vi "iPSread.vi"(8 "error in (no error)":errorcluster, 10 "iPSreadCtrl":T1=enum."Switch Heater Temp", 11 "VISA resource name":refnum<visa-resource-name>) -> (0 "error out":errorcluster, 1 "read buffer":string, 2 "number":dbl, 3 "VISA resource name out":refnum<visa-resource-name>)   [LabVIEW 2017]
uses:
  controls/iPSreadCtrl.ctl
  <vilib>/regexp/Match Regular Expression.xnode
panel:
  out "after match":string
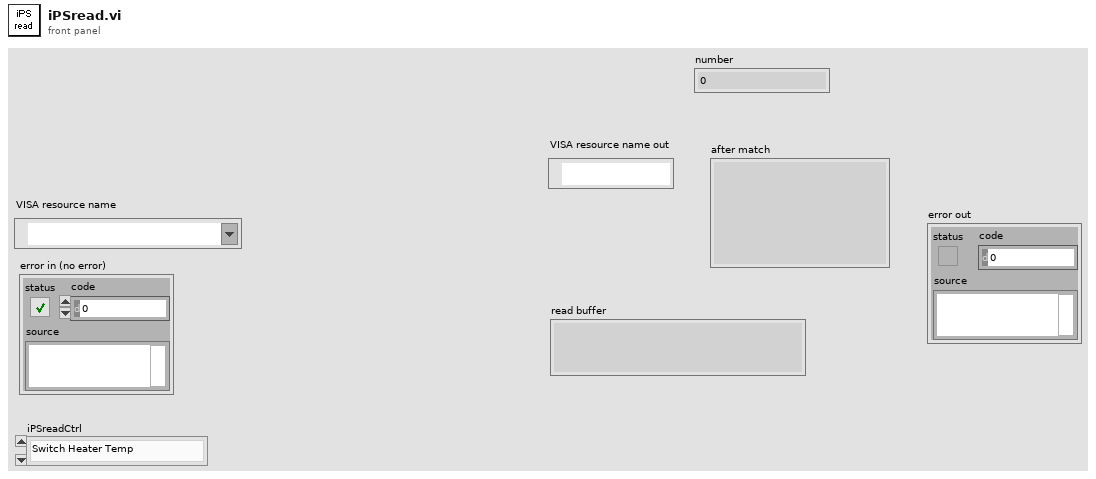
[diagram p1: front panel]
types:
  T1 = typedef "iPSreadCtrl.ctl" = enum16{"OutputField", "MagnetField", "Switch Heater Temp", "Field Rate", "Magnet Temp"}
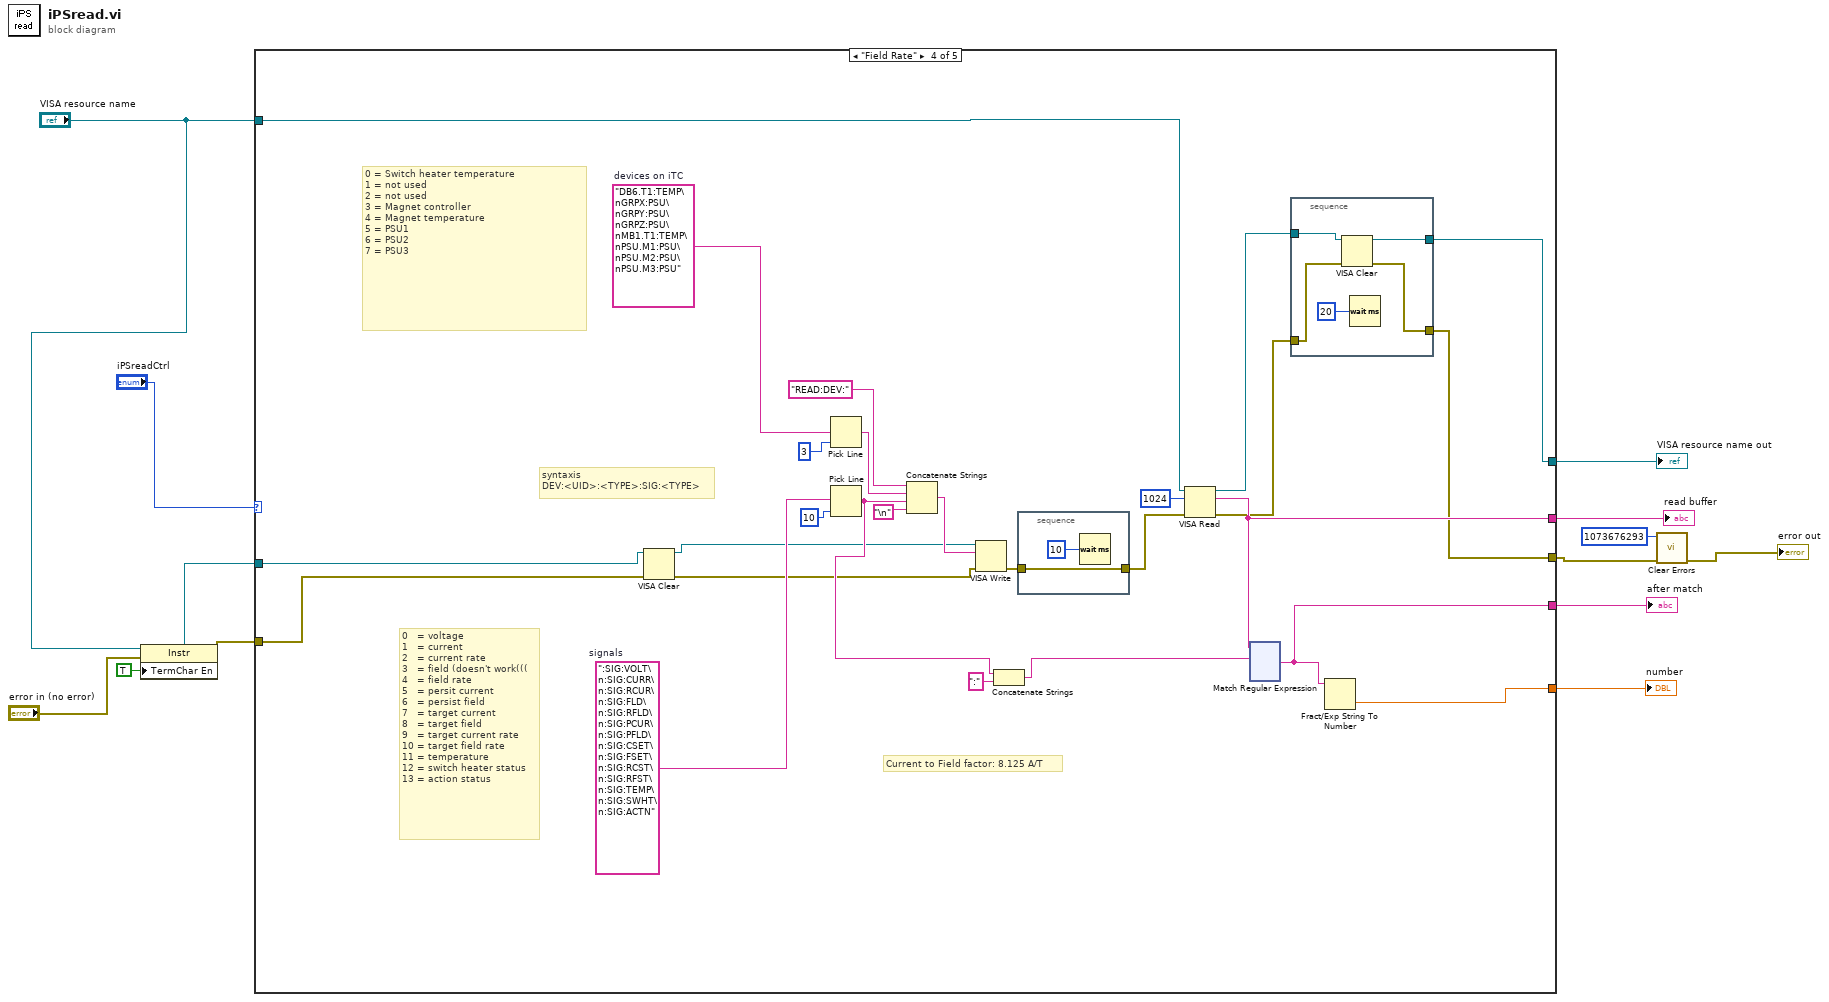
[diagram p0: block diagram]
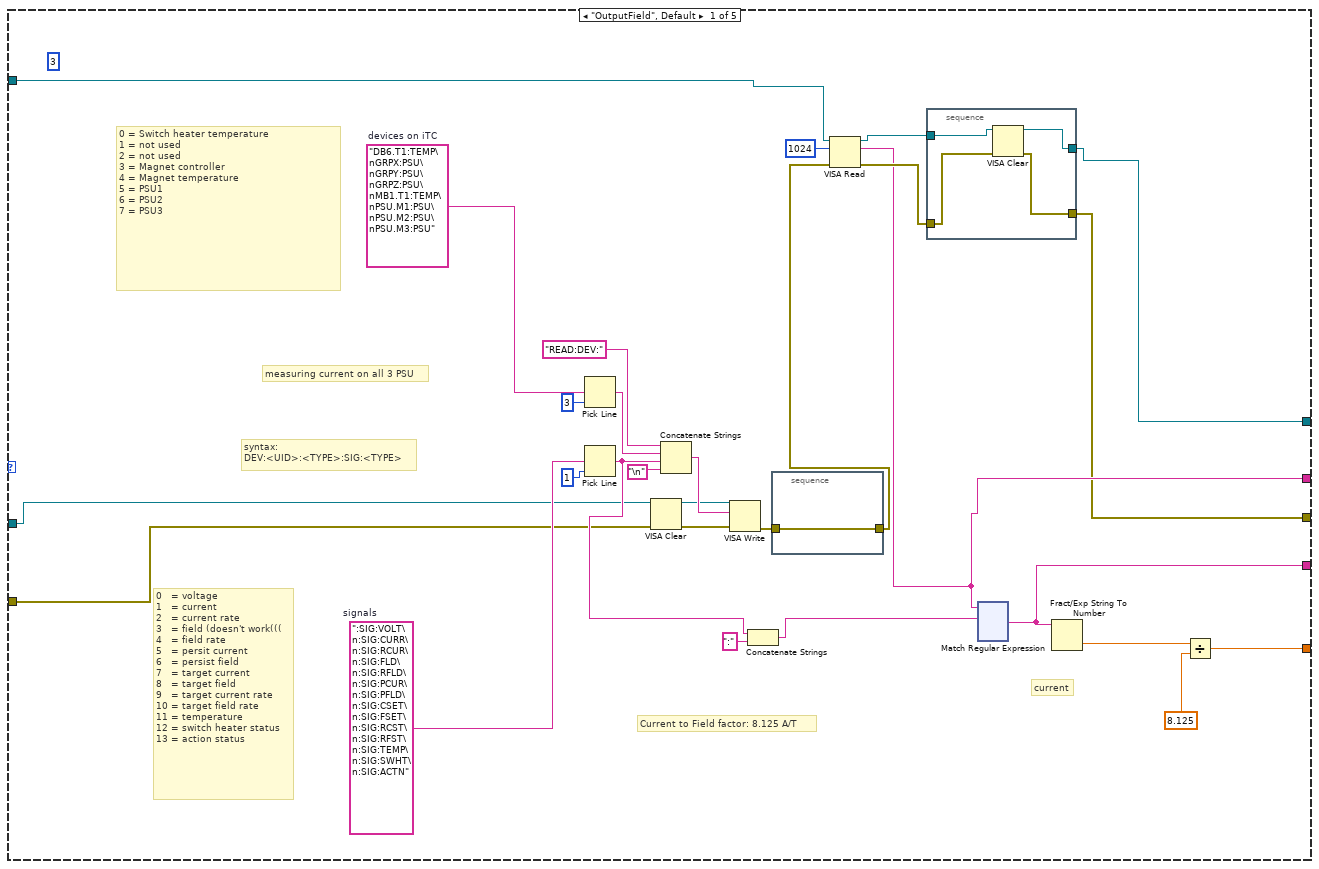
[diagram p2: hidden frame]
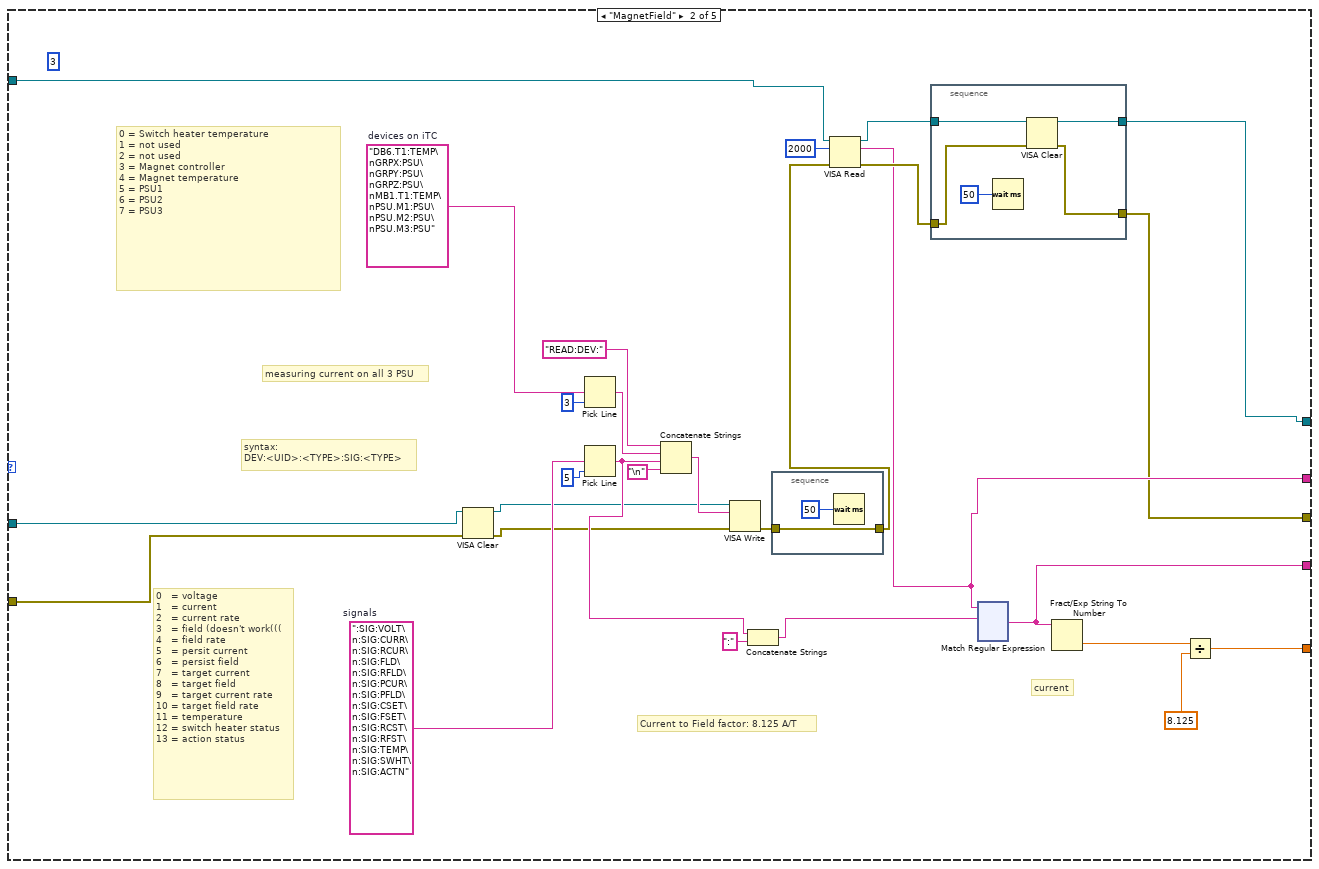
[diagram p3: hidden frame]
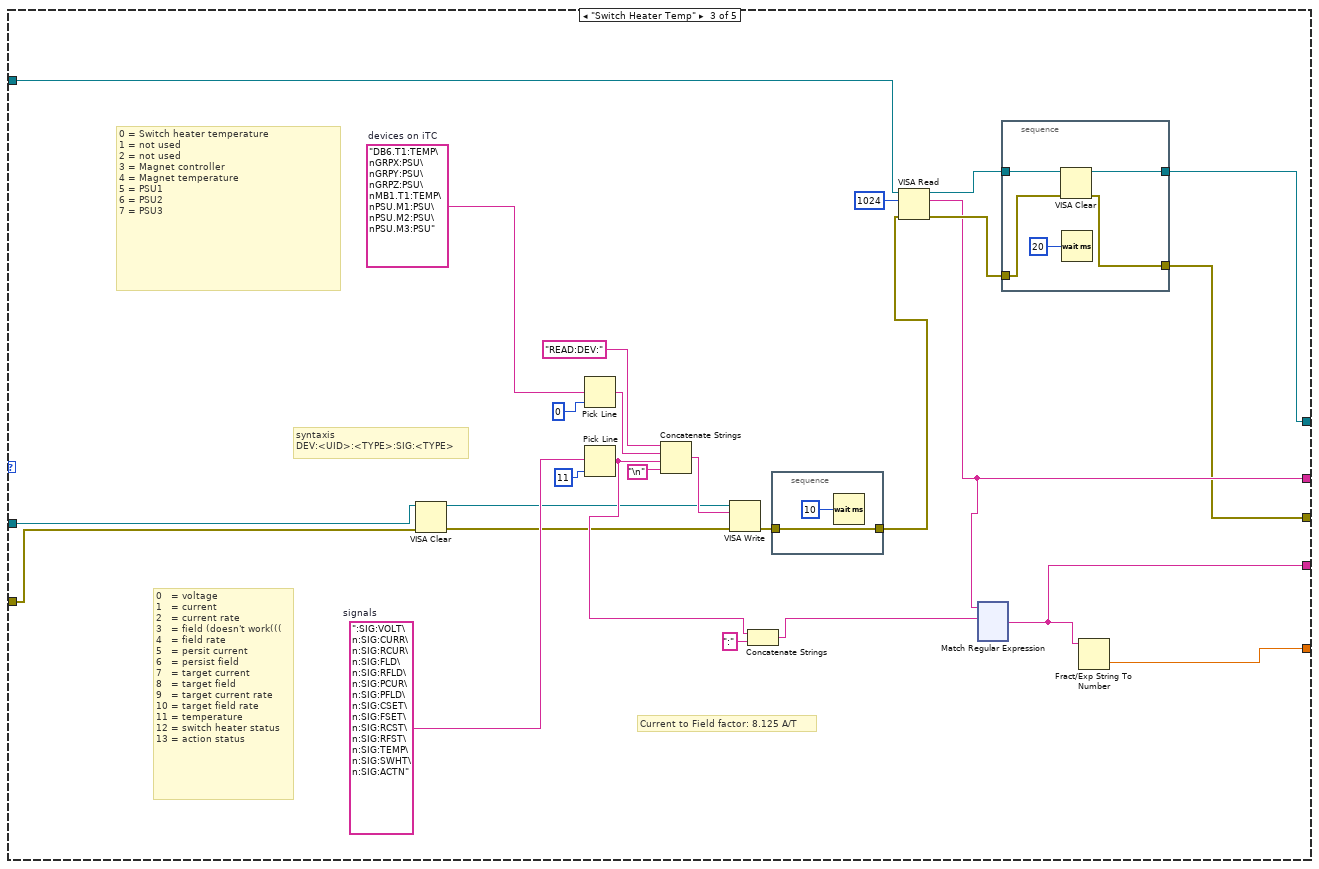
[diagram p4: hidden frame]
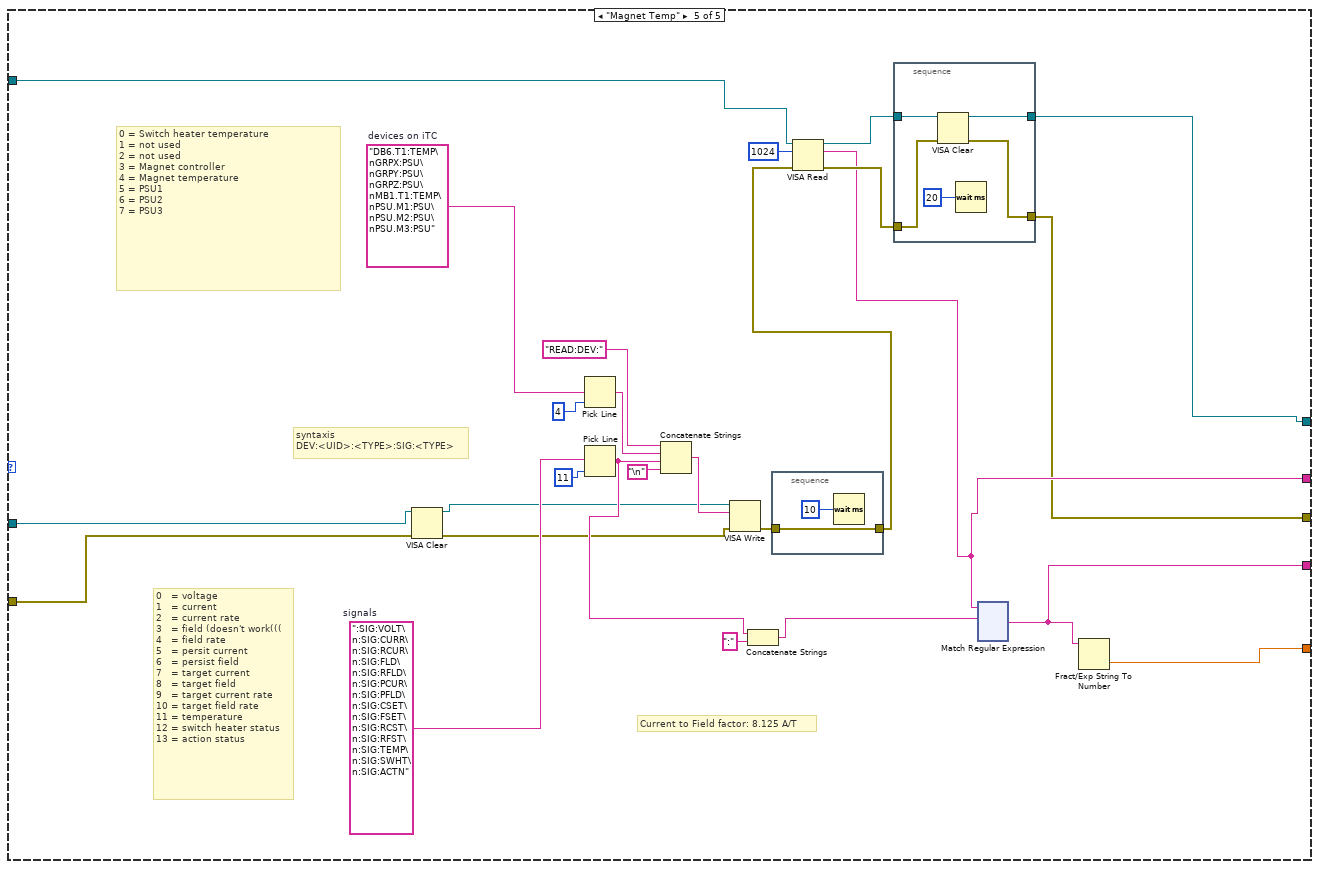
[diagram p5: hidden frame]
diagram:
  n1 = property class="Instr"(reference="VISA resource name", error in="error in (no error)", "TermChar En"=TRUE ("Message Based Settings:Termination Character Enable")) -> (reference out=w7:refnum<visa-resource-name>, error out=w5:errorcluster)
  n2 = case shown="\"Field Rate\"" "iPSreadCtrl" {
    tunnel: "VISA resource name" -> [w20 w164 w310 w454 w601]
    tunnel: [w21 w165 w311 w455 w598] -> w3
    tunnel: [w14 w158 w305 w448 w593] -> w13
    tunnel: [w22 w166 w313 w458 w599] -> w12
    tunnel: [w41 w185 w319 w463 w607] -> w11
    tunnel: [w39 w183 w318 w462 w606] -> w10
    tunnel: w5 -> [w18 w160 w306 w452 w594]
    tunnel: w7 -> [w19 w161 w307 w453 w595]
    frame "OutputField", Default {
      w33 = ":SIG:VOLT\n:SIG:CURR\n:SIG:RCUR\n:SIG:FLD\n:SIG:RFLD\n:SIG:PCUR\n:SIG:PFLD\n:SIG:CSET\n:SIG:FSET\n:SIG:RCST\n:SIG:RFST\n:SIG:TEMP\n:SIG:SWHT\n:SIG:ACTN"  # signals
      w38 = "DB6.T1:TEMP\nGRPX:PSU\nGRPY:PSU\nGRPZ:PSU\nMB1.T1:TEMP\nPSU.M1:PSU\nPSU.M2:PSU\nPSU.M3:PSU"  # devices on iTC
      (unwired) 3
      # "current"
      # "measuring current on all 3 PSU"
      # "Current to Field factor: 8.125 A/T"
      # "0 = Switch heater temperature\n1 = not used\n2 = not used\n3 = Magnet controller \n4 = Magnet temperature\n5 = PSU1 \n6 = PSU2\n7 = PSU3"
      # "0   = voltage\n1   = current\n2   = current rate\n3   = field (doesn't work(((\n4   = field rate\n5   = persit current\n6   = persist field\n7   = target current\n8   = target field\n9   = target current rate\n10 = target field rate \n11 = temperature\n12 = switch heater status\n13 = action status"
      # "syntax:\nDEV:<UID>:<TYPE>:SIG:<TYPE>"
      n3 = Pick Line(multi-line string=w38, line index=3) -> (output string=w35:string)  [unwired: 1 in]
      n4 = Pick Line(multi-line string=w33, line index=1) -> (output string=w31:string)  [unwired: 1 in]
      n5 = VISA Clear(VISA resource name=w19, error in (no error)=w18) -> (VISA resource name out=w17:refnum<visa-resource-name>, error out=w16:errorcluster)
      n6 = Concatenate Strings("READ:DEV:" ("write buffer"), w35, w31, "\n") -> (w29:string)
      n7 = VISA Write(VISA resource name=w17, write buffer=w29, error in (no error)=w16) -> (error out=w37:errorcluster)  [unwired: 2 out]
      n8 = Concatenate Strings(w31, ":" ("string")) -> (w30:string)
      n9 = stacked-sequence {
        tunnel: w37 -> [w157]
        tunnel: [w157] -> w23
        frame #0 {
        }
      }
      n10 = VISA Read(VISA resource name=w20, byte count=u32 1024, error in (no error)=w23) -> (VISA resource name out=w15:refnum<visa-resource-name>, read buffer=w22:string, error out=w24:errorcluster)  [unwired: 1 out]
      n11 = stacked-sequence {
        tunnel: [w44] -> w21
        tunnel: w24 -> [w43]
        tunnel: w15 -> [w42]
        tunnel: [w45] -> w14
        frame #0 {
          n12 = VISA Clear(VISA resource name=w42, error in (no error)=w43) -> (VISA resource name out=w45:refnum<visa-resource-name>, error out=w44:errorcluster)
        }
      }
      n13 = xnode "Match Regular Expression"("input string"=w22, "regular expression"=w30) -> ("after match"=w41:string)  [unwired: 4 in, 4 out]
      n14 = Fract/Exp String To Number(string=w41) -> (number=w26:dbl)  [unwired: 3 in, 1 out]
      n15 = Divide(x=w26, y=8.125) -> (x/y=w39:dbl)
    }
    frame "MagnetField" {
      w177 = ":SIG:VOLT\n:SIG:CURR\n:SIG:RCUR\n:SIG:FLD\n:SIG:RFLD\n:SIG:PCUR\n:SIG:PFLD\n:SIG:CSET\n:SIG:FSET\n:SIG:RCST\n:SIG:RFST\n:SIG:TEMP\n:SIG:SWHT\n:SIG:ACTN"  # signals
      w182 = "DB6.T1:TEMP\nGRPX:PSU\nGRPY:PSU\nGRPZ:PSU\nMB1.T1:TEMP\nPSU.M1:PSU\nPSU.M2:PSU\nPSU.M3:PSU"  # devices on iTC
      (unwired) 3
      # "current"
      # "measuring current on all 3 PSU"
      # "Current to Field factor: 8.125 A/T"
      # "0 = Switch heater temperature\n1 = not used\n2 = not used\n3 = Magnet controller \n4 = Magnet temperature\n5 = PSU1 \n6 = PSU2\n7 = PSU3"
      # "0   = voltage\n1   = current\n2   = current rate\n3   = field (doesn't work(((\n4   = field rate\n5   = persit current\n6   = persist field\n7   = target current\n8   = target field\n9   = target current rate\n10 = target field rate \n11 = temperature\n12 = switch heater status\n13 = action status"
      # "syntax:\nDEV:<UID>:<TYPE>:SIG:<TYPE>"
      n16 = VISA Clear(VISA resource name=w161, error in (no error)=w160) -> (VISA resource name out=w163:refnum<visa-resource-name>, error out=w162:errorcluster)
      n17 = Pick Line(multi-line string=w182, line index=3) -> (output string=w179:string)  [unwired: 1 in]
      n18 = Pick Line(multi-line string=w177, line index=5) -> (output string=w175:string)  [unwired: 1 in]
      n19 = Concatenate Strings("READ:DEV:" ("write buffer"), w179, w175, "\n") -> (w173:string)
      n20 = VISA Write(VISA resource name=w163, write buffer=w173, error in (no error)=w162) -> (error out=w181:errorcluster)  [unwired: 2 out]
      n21 = Concatenate Strings(w175, ":" ("string")) -> (w174:string)
      n22 = stacked-sequence {
        tunnel: w181 -> [w303]
        tunnel: [w303] -> w167
        frame #0 {
          n23 = Wait (ms)(milliseconds to wait=u32 50) -> ()  [unwired: 1 out]
        }
      }
      n24 = VISA Read(VISA resource name=w164, byte count=u32 2000, error in (no error)=w167) -> (VISA resource name out=w159:refnum<visa-resource-name>, read buffer=w166:string, error out=w168:errorcluster)  [unwired: 1 out]
      n25 = stacked-sequence {
        tunnel: [w187] -> w165
        tunnel: w168 -> [w186]
        tunnel: w159 -> [w189]
        tunnel: [w188] -> w158
        frame #0 {
          n26 = Wait (ms)(milliseconds to wait=u32 50) -> ()  [unwired: 1 out]
          n27 = VISA Clear(VISA resource name=w189, error in (no error)=w186) -> (VISA resource name out=w188:refnum<visa-resource-name>, error out=w187:errorcluster)
        }
      }
      n28 = xnode "Match Regular Expression"("input string"=w166, "regular expression"=w174) -> ("after match"=w185:string)  [unwired: 4 in, 4 out]
      n29 = Fract/Exp String To Number(string=w185) -> (number=w170:dbl)  [unwired: 3 in, 1 out]
      n30 = Divide(x=w170, y=8.125) -> (x/y=w183:dbl)
    }
    frame "Switch Heater Temp" {
      w324 = ":SIG:VOLT\n:SIG:CURR\n:SIG:RCUR\n:SIG:FLD\n:SIG:RFLD\n:SIG:PCUR\n:SIG:PFLD\n:SIG:CSET\n:SIG:FSET\n:SIG:RCST\n:SIG:RFST\n:SIG:TEMP\n:SIG:SWHT\n:SIG:ACTN"  # signals
      w329 = "DB6.T1:TEMP\nGRPX:PSU\nGRPY:PSU\nGRPZ:PSU\nMB1.T1:TEMP\nPSU.M1:PSU\nPSU.M2:PSU\nPSU.M3:PSU"  # devices on iTC
      # "Current to Field factor: 8.125 A/T"
      # "0 = Switch heater temperature\n1 = not used\n2 = not used\n3 = Magnet controller \n4 = Magnet temperature\n5 = PSU1 \n6 = PSU2\n7 = PSU3"
      # "0   = voltage\n1   = current\n2   = current rate\n3   = field (doesn't work(((\n4   = field rate\n5   = persit current\n6   = persist field\n7   = target current\n8   = target field\n9   = target current rate\n10 = target field rate \n11 = temperature\n12 = switch heater status\n13 = action status"
      # "syntaxis\nDEV:<UID>:<TYPE>:SIG:<TYPE>"
      n31 = VISA Clear(VISA resource name=w307, error in (no error)=w306) -> (VISA resource name out=w309:refnum<visa-resource-name>, error out=w308:errorcluster)
      n32 = Pick Line(multi-line string=w329, line index=0) -> (output string=w326:string)  [unwired: 1 in]
      n33 = Pick Line(multi-line string=w324, line index=11) -> (output string=w322:string)  [unwired: 1 in]
      n34 = Concatenate Strings("READ:DEV:" ("write buffer"), w326, w322, "\n") -> (w320:string)
      n35 = VISA Write(VISA resource name=w309, write buffer=w320, error in (no error)=w308) -> (error out=w328:errorcluster)  [unwired: 2 out]
      n36 = Concatenate Strings(w322, ":" ("string")) -> (w321:string)
      n37 = stacked-sequence {
        tunnel: w328 -> [w447]
        tunnel: [w447] -> w312
        frame #0 {
          n38 = Wait (ms)(milliseconds to wait=u32 10) -> ()  [unwired: 1 out]
        }
      }
      n39 = VISA Read(VISA resource name=w310, byte count=u32 1024, error in (no error)=w312) -> (VISA resource name out=w304:refnum<visa-resource-name>, read buffer=w313:string, error out=w314:errorcluster)  [unwired: 1 out]
      n40 = xnode "Match Regular Expression"("input string"=w313, "regular expression"=w321) -> ("after match"=w319:string)  [unwired: 4 in, 4 out]
      n41 = stacked-sequence {
        tunnel: [w333] -> w311
        tunnel: w314 -> [w332]
        tunnel: [w331] -> w305
        tunnel: w304 -> [w330]
        frame #0 {
          n42 = VISA Clear(VISA resource name=w330, error in (no error)=w332) -> (VISA resource name out=w331:refnum<visa-resource-name>, error out=w333:errorcluster)
          n43 = Wait (ms)(milliseconds to wait=u32 20) -> ()  [unwired: 1 out]
        }
      }
      n44 = Fract/Exp String To Number(string=w319) -> (number=w318:dbl)  [unwired: 3 in, 1 out]
    }
    frame "Field Rate" {
      w468 = ":SIG:VOLT\n:SIG:CURR\n:SIG:RCUR\n:SIG:FLD\n:SIG:RFLD\n:SIG:PCUR\n:SIG:PFLD\n:SIG:CSET\n:SIG:FSET\n:SIG:RCST\n:SIG:RFST\n:SIG:TEMP\n:SIG:SWHT\n:SIG:ACTN"  # signals
      w473 = "DB6.T1:TEMP\nGRPX:PSU\nGRPY:PSU\nGRPZ:PSU\nMB1.T1:TEMP\nPSU.M1:PSU\nPSU.M2:PSU\nPSU.M3:PSU"  # devices on iTC
      # "Current to Field factor: 8.125 A/T"
      # "0 = Switch heater temperature\n1 = not used\n2 = not used\n3 = Magnet controller \n4 = Magnet temperature\n5 = PSU1 \n6 = PSU2\n7 = PSU3"
      # "0   = voltage\n1   = current\n2   = current rate\n3   = field (doesn't work(((\n4   = field rate\n5   = persit current\n6   = persist field\n7   = target current\n8   = target field\n9   = target current rate\n10 = target field rate \n11 = temperature\n12 = switch heater status\n13 = action status"
      # "syntaxis\nDEV:<UID>:<TYPE>:SIG:<TYPE>"
      n45 = VISA Clear(VISA resource name=w453, error in (no error)=w452) -> (VISA resource name out=w451:refnum<visa-resource-name>, error out=w450:errorcluster)
      n46 = Pick Line(multi-line string=w473, line index=3) -> (output string=w470:string)  [unwired: 1 in]
      n47 = Pick Line(multi-line string=w468, line index=10) -> (output string=w466:string)  [unwired: 1 in]
      n48 = Concatenate Strings("READ:DEV:" ("write buffer"), w470, w466, "\n") -> (w464:string)
      n49 = VISA Write(VISA resource name=w451, write buffer=w464, error in (no error)=w450) -> (error out=w472:errorcluster)  [unwired: 2 out]
      n50 = Concatenate Strings(w466, ":" ("string")) -> (w465:string)
      n51 = stacked-sequence {
        tunnel: w472 -> [w591]
        tunnel: [w591] -> w457
        frame #0 {
          n52 = Wait (ms)(milliseconds to wait=u32 10) -> ()  [unwired: 1 out]
        }
      }
      n53 = VISA Read(VISA resource name=w454, byte count=u32 1024, error in (no error)=w457) -> (VISA resource name out=w449:refnum<visa-resource-name>, read buffer=w458:string, error out=w456:errorcluster)  [unwired: 1 out]
      n54 = xnode "Match Regular Expression"("input string"=w458, "regular expression"=w465) -> ("after match"=w463:string)  [unwired: 4 in, 4 out]
      n55 = stacked-sequence {
        tunnel: [w477] -> w455
        tunnel: w456 -> [w476]
        tunnel: w449 -> [w475]
        tunnel: [w474] -> w448
        frame #0 {
          n56 = VISA Clear(VISA resource name=w475, error in (no error)=w476) -> (VISA resource name out=w474:refnum<visa-resource-name>, error out=w477:errorcluster)
          n57 = Wait (ms)(milliseconds to wait=u32 20) -> ()  [unwired: 1 out]
        }
      }
      n58 = Fract/Exp String To Number(string=w463) -> (number=w462:dbl)  [unwired: 3 in, 1 out]
    }
    frame "Magnet Temp" {
      w612 = ":SIG:VOLT\n:SIG:CURR\n:SIG:RCUR\n:SIG:FLD\n:SIG:RFLD\n:SIG:PCUR\n:SIG:PFLD\n:SIG:CSET\n:SIG:FSET\n:SIG:RCST\n:SIG:RFST\n:SIG:TEMP\n:SIG:SWHT\n:SIG:ACTN"  # signals
      w617 = "DB6.T1:TEMP\nGRPX:PSU\nGRPY:PSU\nGRPZ:PSU\nMB1.T1:TEMP\nPSU.M1:PSU\nPSU.M2:PSU\nPSU.M3:PSU"  # devices on iTC
      # "Current to Field factor: 8.125 A/T"
      # "0 = Switch heater temperature\n1 = not used\n2 = not used\n3 = Magnet controller \n4 = Magnet temperature\n5 = PSU1 \n6 = PSU2\n7 = PSU3"
      # "0   = voltage\n1   = current\n2   = current rate\n3   = field (doesn't work(((\n4   = field rate\n5   = persit current\n6   = persist field\n7   = target current\n8   = target field\n9   = target current rate\n10 = target field rate \n11 = temperature\n12 = switch heater status\n13 = action status"
      # "syntaxis\nDEV:<UID>:<TYPE>:SIG:<TYPE>"
      n59 = VISA Clear(VISA resource name=w595, error in (no error)=w594) -> (VISA resource name out=w597:refnum<visa-resource-name>, error out=w596:errorcluster)
      n60 = Pick Line(multi-line string=w617, line index=4) -> (output string=w614:string)  [unwired: 1 in]
      n61 = Pick Line(multi-line string=w612, line index=11) -> (output string=w610:string)  [unwired: 1 in]
      n62 = Concatenate Strings("READ:DEV:" ("write buffer"), w614, w610, "\n") -> (w608:string)
      n63 = VISA Write(VISA resource name=w597, write buffer=w608, error in (no error)=w596) -> (error out=w616:errorcluster)  [unwired: 2 out]
      n64 = Concatenate Strings(w610, ":" ("string")) -> (w609:string)
      n65 = stacked-sequence {
        tunnel: w616 -> [w735]
        tunnel: [w735] -> w600
        frame #0 {
          n66 = Wait (ms)(milliseconds to wait=u32 10) -> ()  [unwired: 1 out]
        }
      }
      n67 = VISA Read(VISA resource name=w601, byte count=u32 1024, error in (no error)=w600) -> (VISA resource name out=w592:refnum<visa-resource-name>, read buffer=w599:string, error out=w602:errorcluster)  [unwired: 1 out]
      n68 = stacked-sequence {
        tunnel: [w621] -> w598
        tunnel: w602 -> [w620]
        tunnel: [w619] -> w593
        tunnel: w592 -> [w618]
        frame #0 {
          n69 = VISA Clear(VISA resource name=w618, error in (no error)=w620) -> (VISA resource name out=w619:refnum<visa-resource-name>, error out=w621:errorcluster)
          n70 = Wait (ms)(milliseconds to wait=u32 20) -> ()  [unwired: 1 out]
        }
      }
      n71 = xnode "Match Regular Expression"("input string"=w599, "regular expression"=w609) -> ("after match"=w607:string)  [unwired: 4 in, 4 out]
      n72 = Fract/Exp String To Number(string=w607) -> (number=w606:dbl)  [unwired: 3 in, 1 out]
    }
  }
  "read buffer" <- w12
  "VISA resource name out" <- w13
  "after match" <- w11
  "number" <- w10
  n73 = call <vilib>:"Clear Errors.vi"("error in (no error)"=w3, "specific error code to clear (0: all)"=1073676293) -> ("error out"=→"error out":errorcluster)  [unwired: 4 in, 1 out]
